vi "Retrieve Inline Section configuration properties (interactions).vi"(8 "error in":errorcluster, 11 "section item ref in":T2 format="%.0x") -> (0 "error out":errorcluster, 1 "status channel configuration":map{string, map{string, i32}}(c390), 2 "configuration properties":T3[](array[typedef]), 3 "section item ref out":T2 format="%.0x", 4 "Found":bool, 5 "inline vs group data refs":T1 {"item refs - status" format="%.0x"; "item refs - data" format="%.0x"})   [LabVIEW 2019, in "HLA Custom Device System Explorer.lvlib"]
uses:
  HLA Custom Device System Explorer.lvlib
  <vilib>/NI VeriStand/Custom Device API/Custom Device Item Ref.ctl
  Shared/interaction_parameter_configuration.ctl
  Shared/inline_vs_group_refs.ctl
  Shared/Constants.vi
  <vilib>/NI VeriStand/Custom Device API/Get Item Property (String).vi
  <vilib>/NI VeriStand/Custom Device API/Custom Device API.lvlib
  Shared/HLA Custom Device Shared.lvlib
  <vilib>/NI VeriStand/Custom Device Tools/Custom Device Utility Library/Custom Device Utility Library.lvlib
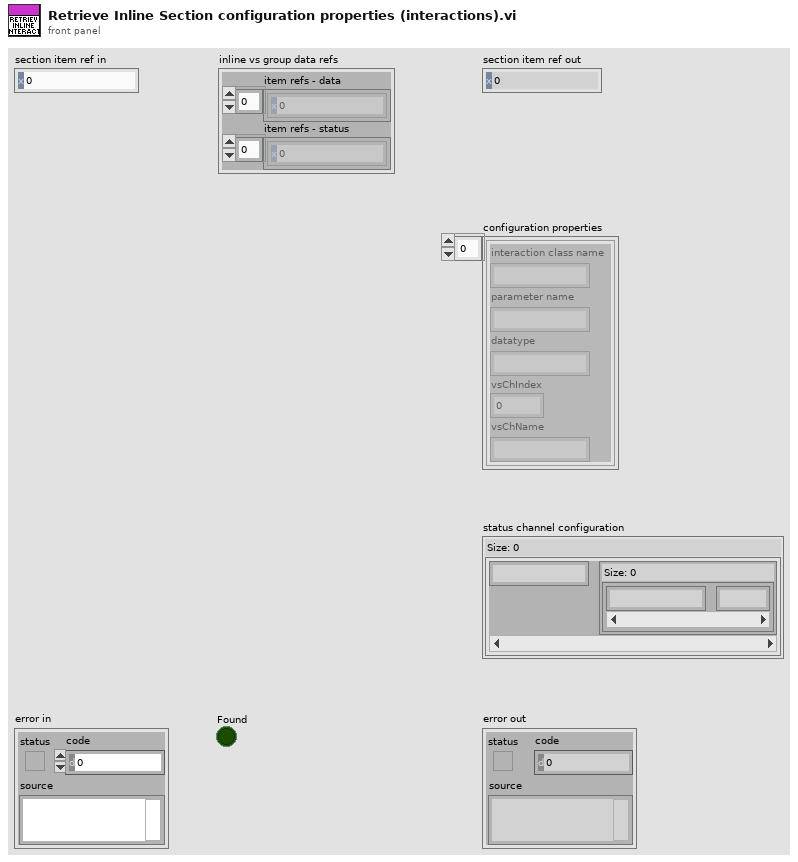
[diagram p1: front panel]
types:
  T1 = typedef "HLA Custom Device Shared.lvlib/inline_vs_group_refs.ctl" = cluster{"item refs - data":T2[], "item refs - status":T2[]}
  T2 = typedef "Custom Device API.lvlib/Custom Device Item Ref.ctl" = u64
  T3 = typedef "HLA Custom Device Shared.lvlib/interaction_parameter_configuration.ctl" = cluster{"interaction class name":string, "parameter name":string, "datatype":string, "vsChIndex":i32, "vsChName":string}
  T4 = typedef "Custom Device API.lvlib/Custom Device Item Info.ctl" = cluster{"Name":string, "Is Channel":bool, "GUID":string, "Is Waveform":bool}
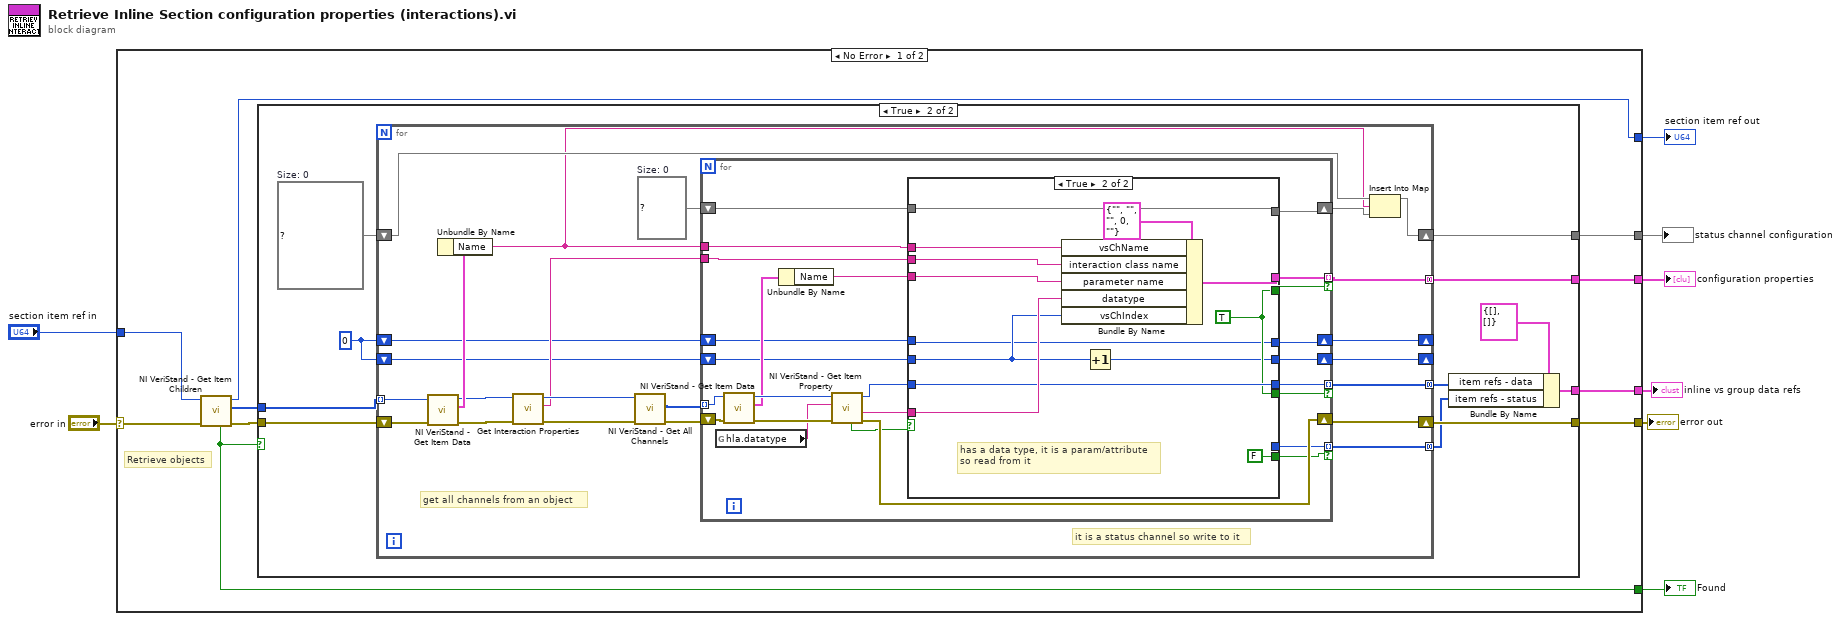
[diagram p0: block diagram]
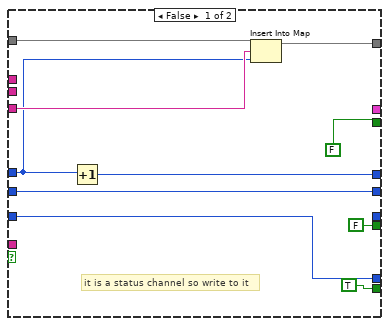
[diagram p3: hidden frame]
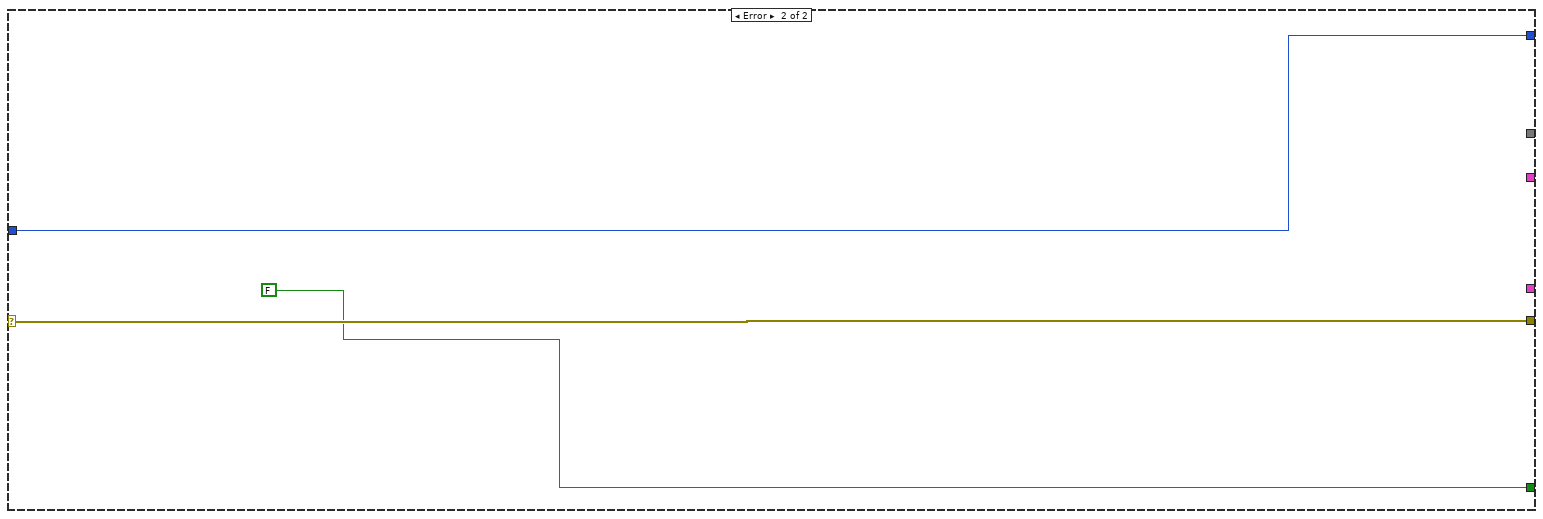
[diagram p4: hidden frame]
diagram:
  n1 = case shown="No Error" "error in" {
    selector: "error in" -> [w15 w103]
    tunnel: [w10 w103] -> w7
    tunnel: [w14 w104] -> w6
    tunnel: "section item ref in" -> [w16 w104]
    tunnel: [w11 FALSE ("Found")] -> w4
    tunnel: [w13 _] -> w3
    tunnel: [w12 _] -> w2
    tunnel: [w9 _] -> w1
    frame No Error {
      # "Retrieve objects"
      n2 = call <vilib>:"NI VeriStand - Get Item Children.vi"("error in (no error)"=w15, "Item Ref in"=w16) -> ("error out"=w17:errorcluster, "Child Refs"=w18:T2[], "Item Ref out"=w14:T2, "Found"=w11:bool)  [unwired: 6 in]
      n3 = case shown="True" w11 {
        tunnel: w18 -> [_ w30]
        tunnel: w17 -> [w19 w29]
        tunnel: [_ w28] -> w13
        tunnel: [_ w26] -> w12
        tunnel: [w19 w24] -> w10
        tunnel: [_ w20] -> w9
        frame False {
        }
        frame True {
          w25 = 0
          w27 = map{string, map{string, i32}} {}  # Size: 0
          n4 = for {
            shift-right: [w45] -> w24
            shift-left: w29 -> [w52]
            tunnel: w30 -> [w51] mode=indexing
            tunnel: [w46] -> w28 mode=concatenating
            shift-right: [w47] -> w26
            shift-left: w27 -> [w49]
            tunnel: [w36] -> w22 mode=concatenating
            tunnel: [w35] -> w21 mode=concatenating
            shift-right: [w32] -> _
            shift-left: w25 -> [w34]
            shift-right: [w31] -> _
            shift-left: w25 -> [w33]
            w50 = map{string, i32} {}  # Size: 0
            # "it is a status channel so write to it"
            # "get all channels from an object"
            n5 = call <vilib>:"NI VeriStand - Get Item Data.vi"("error in (no error)"=w52, "Item Ref in"=w51) -> ("error out"=w42:errorcluster, "Item Info"=w53:T4, "Item Ref out"=w41:T2)  [unwired: 6 in, 1 out]
            n6 = Unbundle By Name(w53) -> ("Name"=w37:string)
            n7 = call "Get Interaction Properties.vi"("error in (no error)"=w42, "Item Ref in"=w41) -> ("error out"=w39:errorcluster, "class name"=w38:string, "Item Ref out"=w40:T2)  [unwired: 7 in]
            n8 = call <vilib>:"NI VeriStand - Get All Channels.vi"("error in"=w39, "Section Ref in"=w40) -> ("error out"=w43:errorcluster, "Channel Refs"=w44:T2[])  [unwired: 6 in, 2 out]
            n9 = for {
              tunnel: w38 -> [w73]
              tunnel: w44 -> [w78] mode=indexing
              tunnel: [w72] -> w46 mode=indexing if=w64
              shift-right: [w71] -> w45
              shift-left: w43 -> [w77]
              shift-right: [w65] -> w48
              shift-left: w50 -> [w66]
              tunnel: w37 -> [w63]
              tunnel: [w61] -> w36 mode=indexing if=w60
              tunnel: [w59] -> w35 mode=indexing if=w58
              shift-right: [w55] -> w32
              shift-left: w34 -> [w57]
              shift-right: [w54] -> w31
              shift-left: w33 -> [w56]
              n10 = global read "Constants.vi" "hla.datatype"() -> (w74:string)
              n11 = call <vilib>:"NI VeriStand - Get Item Data.vi"("error in (no error)"=w77, "Item Ref in"=w78) -> ("error out"=w75:errorcluster, "Item Info"=w69:T4, "Item Ref out"=w76:T2)  [unwired: 6 in, 1 out]
              n12 = Unbundle By Name(w69) -> ("Name"=w68:string)
              n13 = call-poly <vilib>:"NI VeriStand - Get Item Property.vi"("error in (no error)"=w75, "Property Name"=w74, "Item Ref in"=w76) -> ("error out"=w71:errorcluster, "Value"=w70:string, "Item Ref out"=w62:T2, "Found?"=w67:bool)  [unwired: 5 in]
              n14 = case shown="True" w67 {
                tunnel: w73 -> [_ w101]
                tunnel: [_ w100] -> w72
                tunnel: w70 -> [_ w99]
                tunnel: w68 -> [w87 w98]
                tunnel: w66 -> [w88 w97]
                tunnel: [w86 w97] -> w65
                tunnel: [FALSE w93] -> w64
                tunnel: w63 -> [_ w95]
                tunnel: w62 -> [w84 w94]
                tunnel: [_ w94] -> w61
                tunnel: [FALSE w93] -> w60
                tunnel: [w84 _] -> w59
                tunnel: [TRUE FALSE] -> w58
                tunnel: w57 -> [w81 w89]
                tunnel: w56 -> [w79 w91]
                tunnel: [w80 w89] -> w55
                tunnel: [w79 w90] -> w54
                frame False {
                  # "it is a status channel so write to it"
                  n15 = Increment(x=w81) -> (x+1=w80:i32)
                  n16 = Insert Into Map(map in=w88, key=w87, value=w81) -> (map out=w86:map{string, i32})  [unwired: 2 out]
                }
                frame True {
                  w93 = TRUE
                  # "has a data type, it is a param/attribute\nso read from it"
                  n17 = Bundle By Name(cluster=T3 {"interaction class name"="", "parameter name"="", "datatype"="", "vsChIndex"=0, "vsChName"=""}, "vsChName"=w95, "interaction class name"=w101, "parameter name"=w98, "datatype"=w99, "vsChIndex"=w91) -> (w100:T3)
                  n18 = Increment(x=w91) -> (x+1=w90:i32)
                }
              }
            }
            n19 = Insert Into Map(map in=w49, key=w37, value=w48) -> (map out=w47:map{string, map{string, i32}})  [unwired: 2 out]
          }
          n20 = Bundle By Name(cluster=T1 {"item refs - data"=[], "item refs - status"=[]} ("inline vs group data refs"), "item refs - data"=w22, "item refs - status"=w21) -> (w20:T1)
        }
      }
    }
    frame Error {
    }
  }
  "error out" <- w7
  "section item ref out" <- w6
  "Found" <- w4
  "configuration properties" <- w3
  "status channel configuration" <- w2
  "inline vs group data refs" <- w1
